vi "SerialConfig.vi"(1 "Name":string, 2 "flow control":u16(ring) items=["None", "XON/XOFF", "RTS/CTS", "XON/XOFF & RTS/CTS", "DTR/DSR", "XON/XOFF & DTR/DSR"], 3 "stop bits":u16(ring)=20 items=["1.0"=10, "1.5"=15, "2.0"=20], 4 "data bits":u16=8 min=5 max=8 step=1, 5 "baud rate":u32=4000000, 6 "VISA in":refnum<visa-resource-name>) -> (0 "VISA out":refnum<visa-resource-name>)   [LabVIEW 2014]
uses:
  <vilib>/Instr/_visa.llb/VISA Configure Serial Port (Instr).vi
panel:
  in  "end write":bool
  in  "XON Character":u8=17 format="%.0x"
  in  "XOFF Character":u8=19 format="%.0x"
  in  "buffer size":u32=409600
  in  "end read":bool=TRUE
  in  "termination char":u8=10 format="%.0x"
  in  "timeout":u32=1000
  in  "parity":enum16{"None", "Odd", "Even", "Mark", "Space"}(ring)
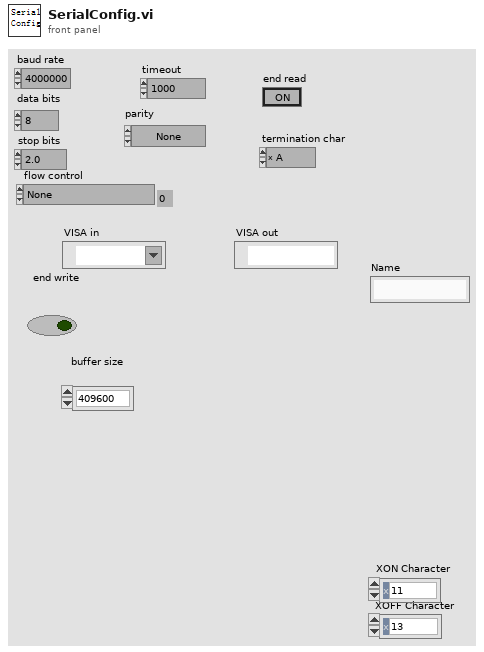
[diagram p1: front panel]
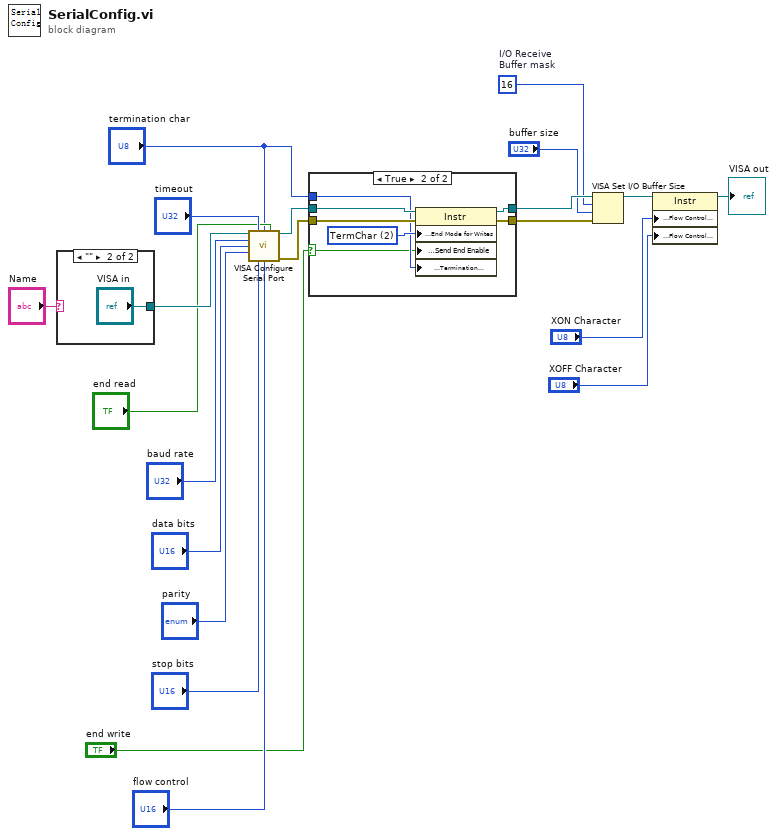
[diagram p0: block diagram]
diagram:
  w5 = u16 16  # I/O Receive Buffer mask
  n1 = case shown="\"\"" "Name" {
    selector: "Name" -> [w22 _]
    tunnel: [w22 "VISA in"] -> w20
    frame Default {
    }
    frame "" {
    }
  }
  n2 = call-poly "VISA Configure Serial Port"("VISA resource name"=w20, "timeout (10sec)"="timeout", "termination char\n(0xA = '\\n' = LF)"="termination char", "Enable Termination\nChar (T)"="end read", "baud rate (9600)"="baud rate", "data bits (8)"="data bits", "parity (0:none)"="parity", "stop bits (10: 1 bit)"="stop bits", "flow control (0:none)"="flow control") -> ("VISA resource name out"=w12:refnum<visa-resource-name>, "error out"=w11:errorcluster)  [unwired: 1 in, 4 out]
  n3 = case shown="True" "end write" {
    selector: "end write" -> [_ w26]
    tunnel: w12 -> [w24 w32]
    tunnel: w11 -> [w25 w31]
    tunnel: [w24 w30] -> w7
    tunnel: [w25 w29] -> w6
    tunnel: "termination char" -> [_ w27]
    frame False {
    }
    frame True {
      w28 = u16 2 items=["None", "LastBit", "TermChar", "Break"] ("Serial Settings:Serial End Mode for Writes")
      n4 = property class="Instr"(reference=w32, error in=w31, "Serial Settings:End Mode for Writes"=w28, "Message Based Settings:Send End Enable"=w26, "Message Based Settings:Termination Character"=w27) -> (reference out=w30:refnum<visa-resource-name>, error out=w29:errorcluster)
    }
  }
  n5 = VISA Set I/O Buffer Size(VISA resource name=w7, mask (16)=w5, size (4096)="buffer size", error in (no error)=w6) -> (VISA resource name out=w9:refnum<visa-resource-name>)  [unwired: 1 out]
  n6 = property class="Instr"(reference=w9, "Serial Settings:Flow Control XON Character"="XON Character", "Serial Settings:Flow Control XOFF Character"="XOFF Character") -> (reference out=→"VISA out":refnum<visa-resource-name>)  [unwired: 1 in, 1 out]
